vi "selectTriggerTest.vi"() -> ()   [LabVIEW 2014]
uses:
  <vilib>/eio/EIONode/EIONode.xnode
  <vilib>/Platform/TimedLoop/XDataNode/XDataNode.xnode
  <vilib>/Platform/TimedLoop/XDataNode/nitl_modes.ctl
  <vilib>/Platform/TimedLoop/XDataNode/XDNodeRunTimeDep.lvlib
  <vilib>/Platform/TimedLoop/XDataNode/wakeup.ctl
  <vilib>/Platform/TimedLoop/XDataNode/timing_clust.ctl
  <vilib>/rvi/eio/common/nirviEmuTemplateMethod_errors.vi
  Controls/selectTrigger.ctl
panel:
  in  "delay(ticks)":u32
  in  "MCSSelectTrigger":T1
  out "Numeric":i32
  in  "stop":bool
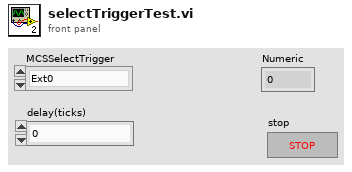
[diagram p1: front panel]
types:
  T1 = typedef "selectTrigger.ctl" = enum8{"Ext0", "Ext1", "Ext2", "Ext3", "Ext4", "Ext5", "Ext6", "Ext7", "Int0", "Int1", "Int2", "Int3", "Int4", "Int5", "Int6", "Int7"}
  T2 = typedef "XDNodeRunTimeDep.lvlib/timing_clust.ctl" = cluster{"Expected End [f-1]":u64, "Actual End [f-1]":u64, "Finished Late? [f-1]":bool, "Expected End [i-1]":u64, "Actual End [i-1]":u64, "Finished Late? [i-1]":bool, "Expected Start [i]":u64, "Actual Start [i]":u64, "Expected Start [f]":u64, "Actual Start [f]":u64, "Source Name":string, "Structure Name":string, "Period":i64, "Deadline":i64, "Offset":i64, "Start":i64, "Priority":i32, "Timeout":i32, "Mode":T3, "Wakeup Reason":T4, "Error":errorcluster, "Source Type":string, "Secondary Source Type":string, "Global End Time":u64, "Global Start Time":u64, "Frame Duration":u64, "Iteration Duration":u64, "Assigned CPU":i32, "I/O Scan Engine Mode":u32}
  T3 = typedef "XDNodeRunTimeDep.lvlib/nitl_modes.ctl" = enum32{"No Change", "Process missed periods, maintain original phase", "Discard missed periods, maintain original phase", "Process missed periods, ignore original phase", "Discard missed periods, ignore original phase"}
  T4 = typedef "XDNodeRunTimeDep.lvlib/wakeup.ctl" = enum32{"Normal", "Aborted", "Asynchronous wakeup", "Timing source error", "Timed loop error", "Timeout"}
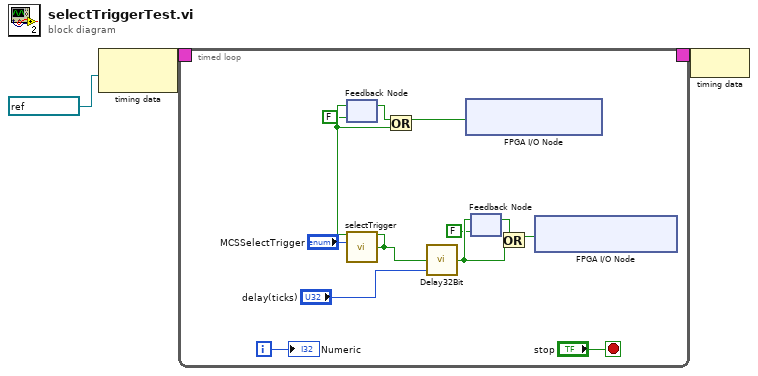
[diagram p0: block diagram]
diagram:
  n1 = node-c288(refnum<k21> "100MHz" ("Source Name")) -> (w3:T2)
  n2 = timed-loop {
    timing: w3 -> [_]
    timing-out: [_] -> w2
    i -> [w14]
    stop <- "stop" stop-if-true
    n3 = feedback #1(FALSE ("risEdge")) -> (w9:bool)
    n4 = call "selectTrigger.vi"("MCSSelectTrigger"="MCSSelectTrigger") -> ("fired"=w10:bool)  [unwired: 4 in]
    n5 = feedback-in #1(w10) -> ()
    n6 = Or(x=w9, y=w10) -> (x .or. y?=w11:bool)
    n7 = call "Delay32Bit.vi"("delay(ticks)"="delay(ticks)", "In"=w10) -> ("Out"=w7:bool)  [unwired: 3 in]
    n8 = xnode "FPGA I/O Node"("Connector1/DIO5"=w11) -> ()  [unwired: 1 in, 1 out]
    n9 = feedback #2(FALSE ("Out")) -> (w5:bool)
    n10 = feedback-in #2(w7) -> ()
    n11 = Or(x=w5, y=w7) -> (x .or. y?=w6:bool)
    n12 = xnode "FPGA I/O Node"("Connector1/DIO12"=w6) -> ()  [unwired: 1 in, 1 out]
    "Numeric" <- w14
  }
  n13 = node-c288(w2) -> ()
